vi "up hole Pressure 2016.vi"(0 "Sensor Cluster":T1, 1 "Pressure Offset":dbl format="%.2f", 2 "Array in":refnum<k24>[](array[refnum]), 5 "Pressure \nSlope":dbl=24.27199935913086 format="%.2f", 7 "Descriptions":string[](array[string]), 9 "Zero Pressure\n(F = leave as is)":bool) -> (3 "Array out":refnum<k24>[](array[refnum]), 4 "Uphole Pressure":dbl format="%.2f", 13 "Sensor Cluster 2":T1)   [LabVIEW 2016]
uses:
  Waterloo DAQ/controls/MCC DAQ Readings.ctl
  C:/Program Files (x86)/National Instruments/LabVIEW 2016/vi.lib/ULx/ULx_LV.dll
panel:
  out "Voltage":dbl format="%.2f"
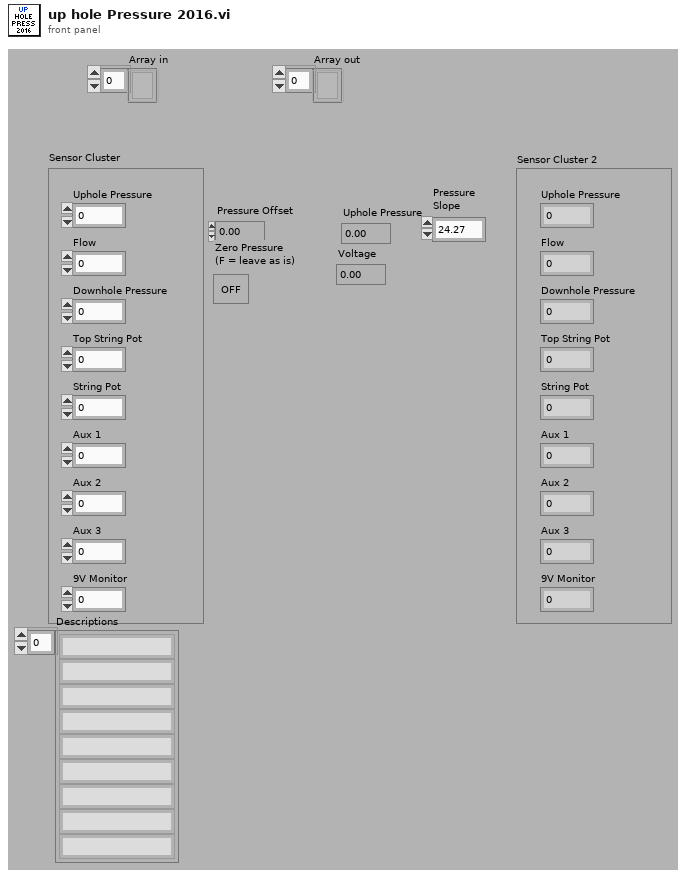
[diagram p1: front panel]
types:
  T1 = typedef "MCC DAQ Readings.ctl" = cluster{"Uphole Pressure":dbl, "Flow":dbl, "Downhole Pressure":dbl, "Top String Pot":dbl, "String Pot":dbl, "Aux 1":dbl, "Aux 2":dbl, "Aux 3":dbl, "9V Monitor":dbl}
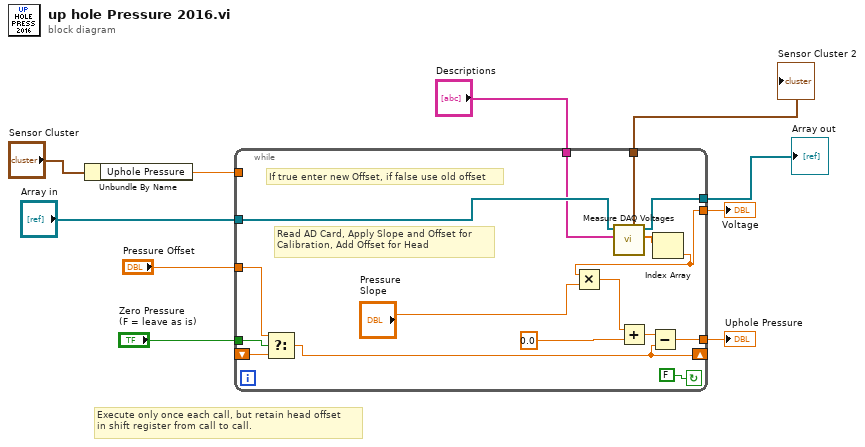
[diagram p0: block diagram]
diagram:
  # "Execute only once each call, but retain head offset \nin shift register from call to call."
  n1 = Unbundle By Name("Sensor Cluster") -> ("Uphole Pressure"=w6:dbl)
  n2 = while {
    tunnel: "Zero Pressure\n(F = leave as is)" -> [w22]
    tunnel: "Pressure Offset" -> [w23]
    shift-left: _ -> [w24]
    shift-right: [w18] -> _
    tunnel: [w21] -> w10
    tunnel: [w11] -> w7
    tunnel: w6 -> [_]
    tunnel: "Array in" -> [w16]
    tunnel: [w15] -> w4
    tunnel: [w14] -> w2
    tunnel: "Descriptions" -> [w12]
    stop <- FALSE continue-if-true
    # "Read AD Card, Apply Slope and Offset for\nCalibration, Add Offset for Head"
    # "If true enter new Offset, if false use old offset"
    n3 = Select(t=w23, s=w22, f=w24) -> (s? t:f=w18:dbl)
    n4 = call "Measure DAQ Voltages.vi"("Descriptions"=w12, "Array in"=w16) -> ("Raw Voltages"=w13:dbl[], "Array out"=w15:refnum<k24>[], "Sensor Cluster"=w14:T1)  [unwired: 7 in]
    n5 = Index Array(array=w13) -> (element=w11:dbl)  [unwired: 1 in]
    n6 = Multiply(x=w11, y="Pressure \nSlope") -> (x*y=w26:dbl)
    n7 = Add(x=w26, y=0.0 ("Offset")) -> (x+y=w19:dbl)
    n8 = Subtract(x=w19, y=w18) -> (x-y=w21:dbl)
  }
  "Uphole Pressure" <- w10
  "Voltage" <- w7
  "Array out" <- w4
  "Sensor Cluster 2" <- w2
